vi "Write Message.vi"(10 "Message":string, 11 "IAction in":refnum<class "IAction.lvclass">) -> (3 "IAction out":refnum<class "IAction.lvclass">)   [LabVIEW 2019, in "IAction.lvclass"]
uses:
  IAction.lvclass
  IAction.lvclass/IAction.ctl
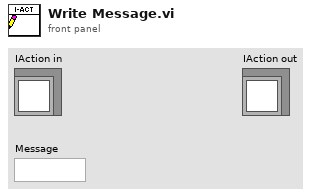
[diagram p1: front panel]
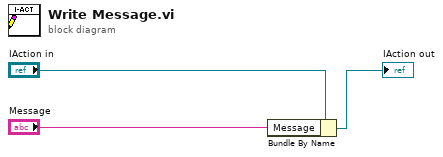
[diagram p0: block diagram]
diagram:
  n1 = Bundle By Name(cluster="IAction in", "Message"="Message") -> (→"IAction out":refnum<class "IAction.lvclass">)
